vi "Initialize.vi"(8 "error in":errorcluster, 11 "Masterflex 75211 Settings":T1) -> (0 "error out":errorcluster, 1 "Initialized":bool, 3 "Masterflex 75211 Settings":T1)   [LabVIEW 2021, in "Masterflex 75211.lvlib"]
uses:
  Masterflex 75211.lvlib
  Masterflex 75211 DAQ Setting.ctl
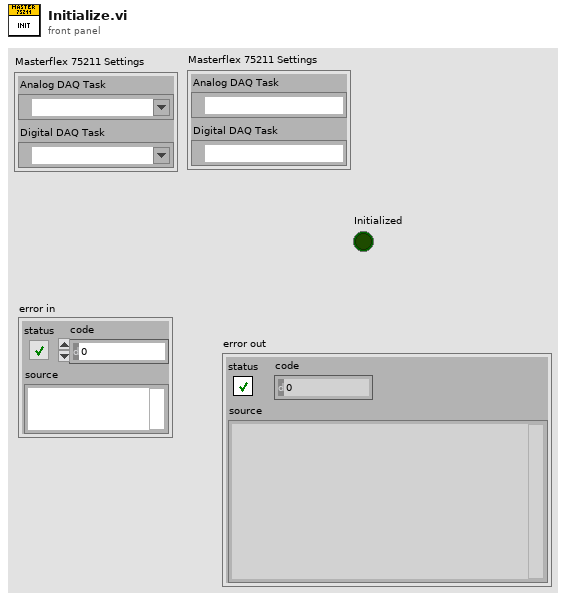
[diagram p1: front panel]
types:
  T1 = typedef "Masterflex 75211.lvlib/Masterflex 75211 DAQ Setting.ctl" = cluster{"Analog DAQ Task":refnum<k21>, "Digital DAQ Task":refnum<k21>}
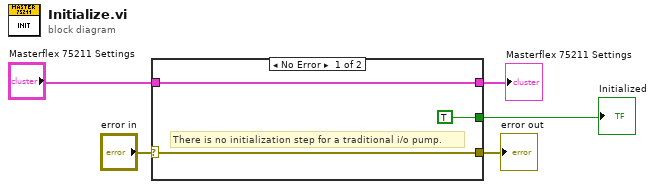
[diagram p0: block diagram]
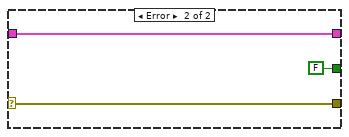
[diagram p2: hidden frame]
diagram:
  n1 = case shown="No Error" "error in" {
    selector: "error in" -> [w8 w10]
    tunnel: [w8 w10] -> w4
    tunnel: "Masterflex 75211 Settings" -> [w7 w11]
    tunnel: [w7 w11] -> w1
    tunnel: [TRUE ("Initialized") FALSE ("Initialized")] -> w3
    frame No Error {
      # "There is no initialization step for a traditional i/o pump."
    }
    frame Error {
    }
  }
  "error out" <- w4
  "Initialized" <- w3
  "Masterflex 75211 Settings" <- w1
